vi "MotionProfiling_1D_ExampleSchedualingLoop.vi"(8 "error in (no error)":errorcluster, 10 "MotorName":string="DUT", 11 "file path (dialog if empty)":path=path "/home/lvuser/mp3.csv") -> (0 "error out":errorcluster)   [LabVIEW 2017]
panel:
  out "Loop Time":u32(knob) scale=0.0..20.0
  out "Velocity":i32(graph)
  out "Position":i32(graph)
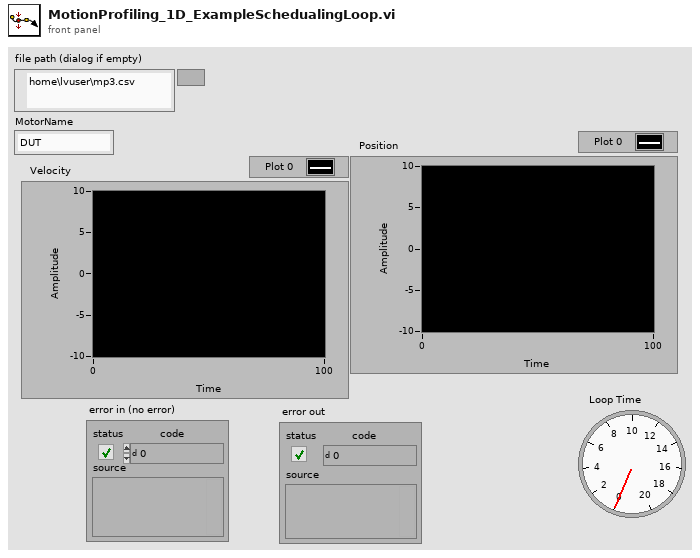
[diagram p1: front panel]
types:
  T1 = typedef "WPI_MotorControlDeviceRef.ctl" = cluster{"DeviceStatus":errorcluster, "Type":T2, "PWM":cluster{"PWM Channel":T3, "DeadBand":T4}, "CAN":cluster{"Device Number":u8, "SetOutput VI Ref":variant, "GetOutput VI Ref":variant, "Enable VI Ref":variant, "Disable VI Ref":variant, "Data":variant}, "Invert":bool, "DIO PWM":cluster{"PWM \"Enable\" Channel":T3, "DIOChannel":T5, "PWM Rate":dbl}}
  T2 = typedef "WPI_MotorControlType.ctl" = enum16{"PWM", "CAN", "DIO PWM"}
  T3 = typedef "FPGA_DIOPWMChannel.ctl" = enum8{"PWM 0", "PWM 1", "PWM 2", "PWM 3", "PWM 4", "PWM 5", "PWM 6", "PWM 7", "PWM 8", "PWM 9", "PWM MXP 0", "PWM MXP 1", "PWM MXP 2", "PWM MXP 3", "PWM MXP 4", "PWM MXP 5", "PWM MXP 6", "PWM MXP 7", "PWM MXP 8", "PWM MXP 9", "Invalid"}
  T4 = typedef "WPI_PWMDeadband.ctl" = cluster{"Name":string, "maxPositivePwm":i32, "minPositivePwm":i32, "centerPwm":i32, "maxNegativePwm":i32, "minNegativePwm":i32, "angularRange":u16}
  T5 = typedef "FPGA_DIOChannel.ctl" = enum8{"DIO 0", "DIO 1", "DIO 2", "DIO 3", "DIO 4", "DIO 5", "DIO 6", "DIO 7", "DIO 8", "DIO 9", "DIO MXP 0", "DIO MXP 1", "DIO MXP 2", "DIO MXP 3", "DIO MXP 4", "DIO MXP 5", "DIO MXP 6", "DIO MXP 7", "DIO MXP 8", "DIO MXP 9", "DIO MXP 10", "DIO MXP 11", "DIO MXP 12", "DIO MXP 13", "DIO MXP 14", "DIO MXP 15", "SPI Port CS1", "SPI Port CS2", "SPI Port CS3", "SPI Port MISO", "SPI Port MOSI", "Invalid"}
  T6 = cluster{"Top Buffer Remaining":i32, "Top Buffer Count":i32, "Bottom Buffer Count":i32, "Has Underrun?":bool, "Is Underrun?":bool, "Active Point Valid?":bool, "Is Last?":bool, "Profile Slot Select 0":i32, "Output Enable":i32, "Time Duration (ms)":i32, "Profile Slot Select 1":i32}
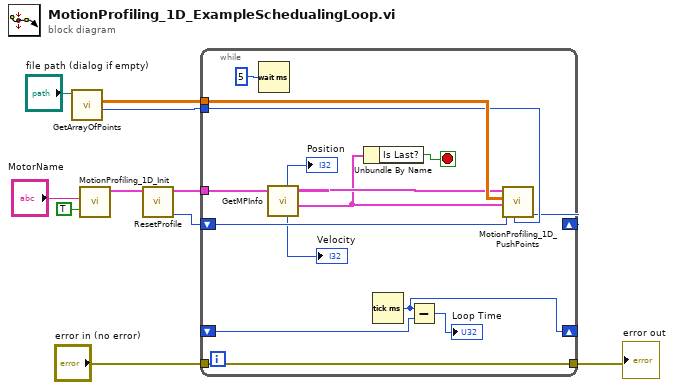
[diagram p0: block diagram]
diagram:
  n1 = call "GetArrayOfPoints.vi"("file path (dialog if empty)"="file path (dialog if empty)") -> ("Number of Points"=w3:i32, "Array of Trajectory Points"=w4:dbl[][])  [unwired: 9 in]
  n2 = call "MotionProfiling_1D_Init.vi"("Zero Sensor?"=TRUE, "MotorName"="MotorName") -> ("PhoenixMotorControlDevRef"=w7:T1)  [unwired: 9 in]
  n3 = call "ResetProfile.vi"("PhoenixMotorControlDevRef"=w7) -> ("CursorOut"=w5:u32, "PhoenixMotorControlDevRef Out"=w6:T1)  [unwired: 9 in]
  n4 = while {
    tunnel: w6 -> [w21]
    shift-right: [w19] -> _
    shift-left: w5 -> [w23]
    tunnel: w4 -> [w24]
    tunnel: w3 -> [w22]
    tunnel: [w14] -> w2
    tunnel: "error in (no error)" -> [w14]
    shift-right: [w13] -> _
    shift-left: _ -> [w12]
    stop <- w15 stop-if-true
    n5 = Wait (ms)(milliseconds to wait=u32 5) -> ()  [unwired: 1 out]
    n6 = call "GetMPInfo.vi"("PhoenixMotorControlDevRef"=w21) -> ("Motion Profile Status"=w16:T6, "PhoenixMotorControlDevRef Out"=w20:T1, "Velocity (Sensor Units per 100 ms)"=→"Velocity":i32, "Position (Sensor Units)"=→"Position":i32)  [unwired: 5 in, 2 out]
    n7 = Unbundle By Name(w16) -> ("Is Last?"=w15:bool)
    n8 = Tick Count (ms)() -> (millisecond timer value=w13:u32)
    n9 = Subtract(x=w13, y=w12) -> (x-y=→"Loop Time":u32)
    n10 = call "MotionProfiling_1D_PushPoints.vi"("NumberOfPoints"=w22, "CursorIn"=w23, "Motion Profile Status"=w16, "ArrayOfTrajectoyPoints"=w24, "PhoenixMotorControlDevRef"=w20) -> ("CursorOut"=w19:u32)  [unwired: 5 in, 1 out]
  }
  "error out" <- w2
